vi "5001 Step Type Not Supported.vi"(8 "error in (no error)":errorcluster, 11 "Step Type":string) -> (0 "error out":errorcluster)   [LabVIEW 2020, in "MacroAssert.lvlib" / "Custom Errors.lvlib"]
uses:
  Custom Errors.lvlib
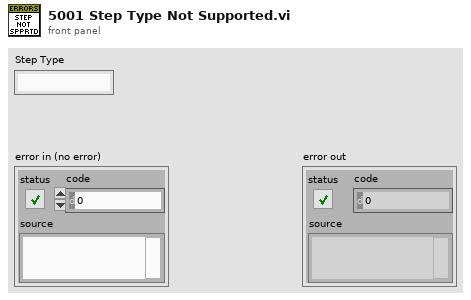
[diagram p1: front panel]
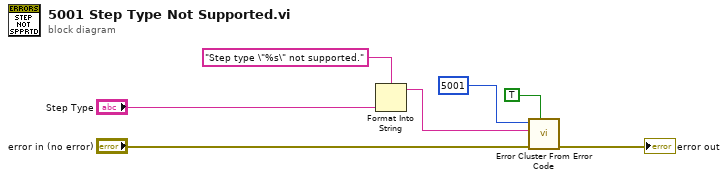
[diagram p0: block diagram]
diagram:
  n1 = Format Into String(format string="Step type \"%s\" not supported.", "Step Type") -> (resulting string=w3:string)  [unwired: 2 in, 1 out]
  n2 = call <vilib>:"Error Cluster From Error Code.vi"("show call chain? (False)"=TRUE, "error in (no error)"="error in (no error)", "error message (\"\")"=w3, "error code (0)"=5001) -> ("error out"=→"error out":errorcluster)  [unwired: 5 in]
